vi "Subpanel Listening Server.vi"(8 "error in (no error)":errorcluster, 11 "Plugin in":refnum<class "Generic Plugin.lvclass">) -> (0 "error out":errorcluster, 3 "Plugin out":refnum<class "Generic Plugin.lvclass">)   [LabVIEW 2020, in "Generic Plugin.lvclass"]
doc: "Listening server VI that will listen to the assigned Receiving Queue of the object, which is receiving messages from a plugin. The Listening Server Cases VI should be overridden and updated to properly respond to messages from a plugin."
uses:
  Generic Plugin.lvclass
  Generic Plugin.lvclass/Generic Plugin.ctl
  <userlib>/Dynamic Reentrant/Type Defs/Message.ctl
  <userlib>/Dynamic Reentrant/Dynamic Reentrant.lvlib
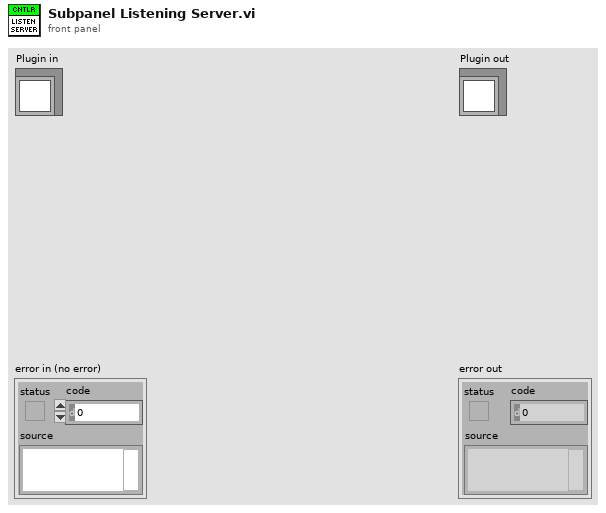
[diagram p1: front panel]
types:
  T1 = typedef "Dynamic Reentrant.lvlib/Message.ctl" = cluster{"Source":string, "Destination":string, "Time Stamp":timestamp, "Command":string, "Data":variant}
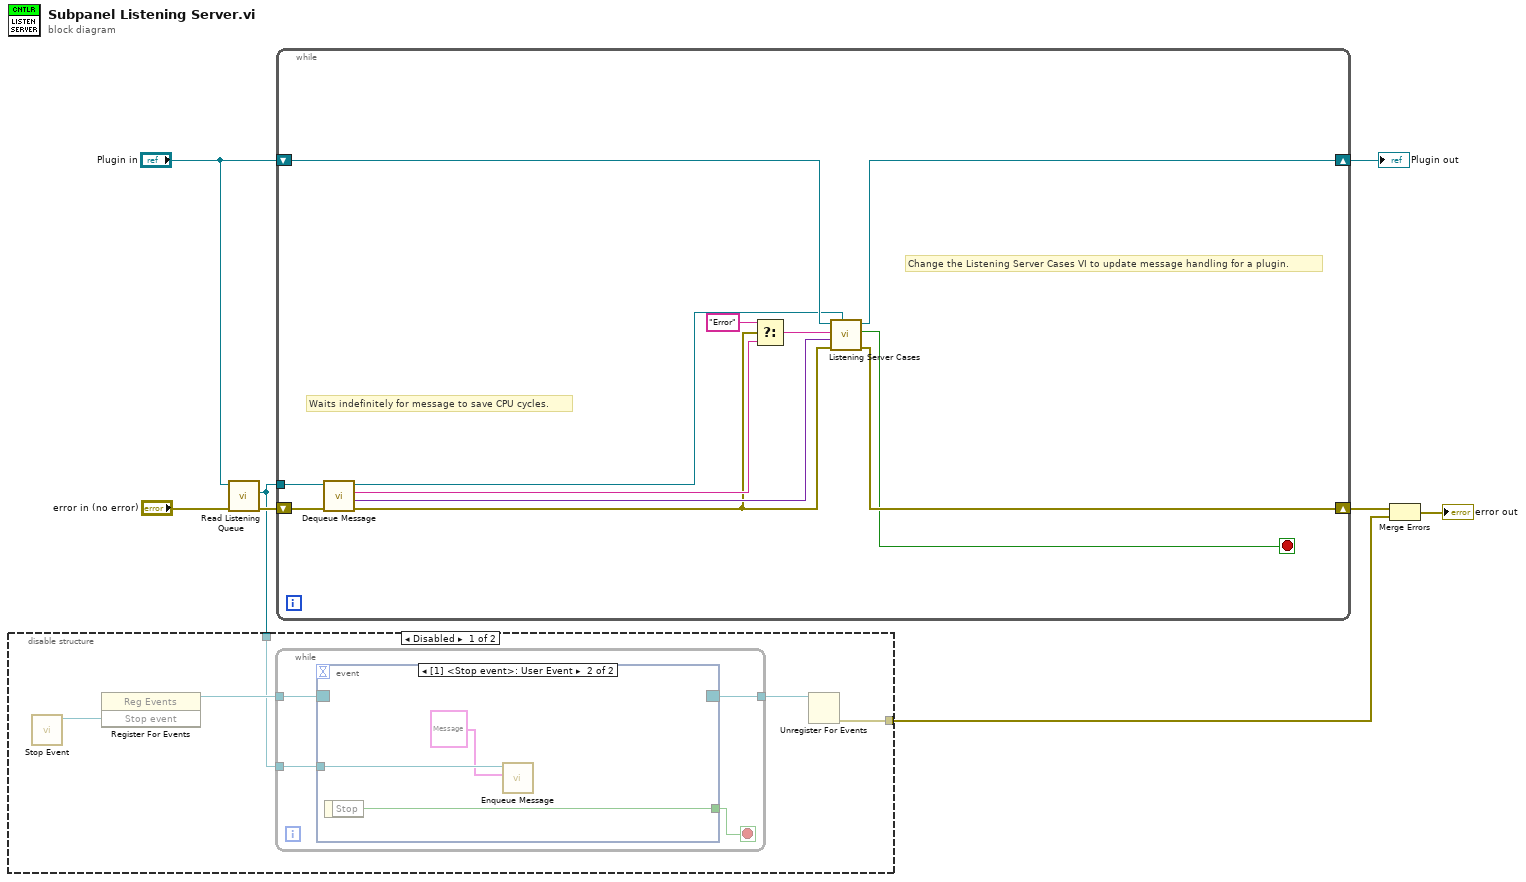
[diagram p0: block diagram]
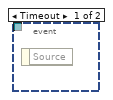
[diagram p2: hidden frame]
diagram:
  n1 = call "Read Listening Queue.vi"("error in (no error)"="error in (no error)", "Generic Controller in"="Plugin in") -> ("error out"=w5:errorcluster, "Listening Queue"=w4:refnum<queue>)  [unwired: 7 in, 1 out]
  n2 = disable-structure shown="Disabled" {
    disable-tunnel: w4 -> [w10 _]
    disable-tunnel: [w9 _] -> w2
    frame Disabled {
      n3 = call "Stop Event.vi"() -> ("Stop event"=w12:refnum<user-event>)  [unwired: 11 in]
      n4 = register-events(w12) -> (reference out=w11:refnum<event-registration>)  [unwired: 2 in, 1 out]
      n5 = while {
        tunnel: w10 -> [w17]
        tunnel: w11 -> [w16]
        tunnel: [w15] -> w13
        stop <- w14 stop-if-true
        n6 = event shown="[1] <Stop event>: User Event" {
          selector: w16 -> [_ _]
          dyn-events: [_ _] -> w15
          timeout: _ -> [_ _]
          tunnel: w17 -> [_ w19]
          tunnel: [_ w20] -> w14
          event Timeout {
            n7 = event-data() -> ()  [unwired: 1 in, 1 out]
          }
          event User Event {
            n8 = event-data() -> ("Stop"=w20:bool)  [unwired: 1 in]
            n9 = call <userlib>:"Enqueue Message.vi"("Message"=T1 {"Source"="", "Destination"="", "Time Stamp"=timestamp(0 s since 1904-01-01), "Command"="Exit", "Data"=variant(string "")}, "Listening Queue"=w19) -> ()  [unwired: 8 in, 2 out]
          }
        }
      }
      n10 = Unregister For Events(event registration refnum=w13) -> (error out=w9:errorcluster)  [unwired: 1 in]
    }
    frame Enabled {
    }
  }
  n11 = while {
    shift-right: [w32] -> w8
    shift-left: w5 -> [w29]
    shift-right: [w31] -> w1
    shift-left: "Plugin in" -> [w30]
    tunnel: w4 -> [w28]
    stop <- w26 stop-if-true
    # "Waits indefinitely for message to save CPU cycles."
    # "Change the Listening Server Cases VI to update message handling for a plugin."
    n12 = call <userlib>:"Dequeue Message.vi"("error in (no error)"=w29, "Listening Queue"=w28) -> ("error out"=w21:errorcluster, "Data"=w27:variant, "Command"=w24:string, "queue out"=w25:refnum<queue>)  [unwired: 2 in, 4 out]
    n13 = Select(t="Error", s=w21, f=w24) -> (s? t:f=w23:string)
    n14 = call-dynamic "Listening Server Cases.vi"("Listening Queue"=w25, "error in (no error)"=w21, "Data"=w27, "Command"=w23, "Generic Controller in"=w30) -> ("error out"=w32:errorcluster, "Stop?"=w26:bool, "Generic Controller out"=w31:refnum<class "Generic Plugin.lvclass">)  [unwired: 4 in]
  }
  "Plugin out" <- w1
  n15 = Merge Errors(w8, w2) -> (→"error out":errorcluster)
